vi "multiplier color to multiplier value.vi"(2 "mult color":T1) -> (6 "multiplier":dbl)   [LabVIEW 2018]
uses:
  multiplier--control.ctl
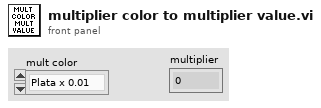
[diagram p1: front panel]
types:
  T1 = typedef "multiplier--control.ctl" = enum16{"Plata x 0.01", "Oro x 0.1 ", "Negro - x 1", "Marrón - x 10", "Rojo - x 100", "Naranja - x 1k", "Amarillo - x 10k", "Verde - 100k", "Azul - x 1M", "Violeta - x10 M", "Gris - x 100M", "Blanco - x 1G"}
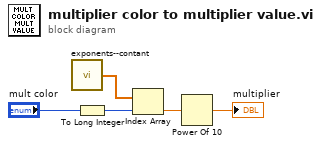
[diagram p0: block diagram]
diagram:
  n1 = call "exponents--contant.vi"() -> ("exponent"=w3:dbl[])  [unwired: 6 in]
  n2 = To Long Integer(number="mult color") -> (32bit integer=w4:i32)
  n3 = Index Array(array=w3, index=w4) -> (element=w2:dbl)
  n4 = Power Of 10(x=w2) -> (10^x=→"multiplier":dbl)
